vi "makeBlankPic.vi"(7 "File Path":path, 11 "previousImageData":T2) -> (1 "bottom":i16, 2 "right":i16, 3 "missingPicture":picture)   [LabVIEW 2022 SP3]
uses:
  <vilib>/picture/picture.llb/imagedata.ctl
  TOAPspecs.ctl
panel:
  in  "TOAPspecs":T1={"textOrigin"={"x"=0, "y"=0}, "textAlignment"={"horizontal"=enum."center", "vertical"=enum."center"}, "fontColour"={"text color"=16448250, "BG color"=1132933, "orientation "=enum."None"}, "fontChoice"=enum."User-specified Font", "userFont"={"Font Name:"="Courier New", "Size"=14, "Strikeout?"=FALSE, "Italic?"=FALSE, "Underline?"=FALSE, "Outline?"=FALSE, "Shadow?"=FALSE, "Bold?"=FALSE}}
  out "missingImageData":T2
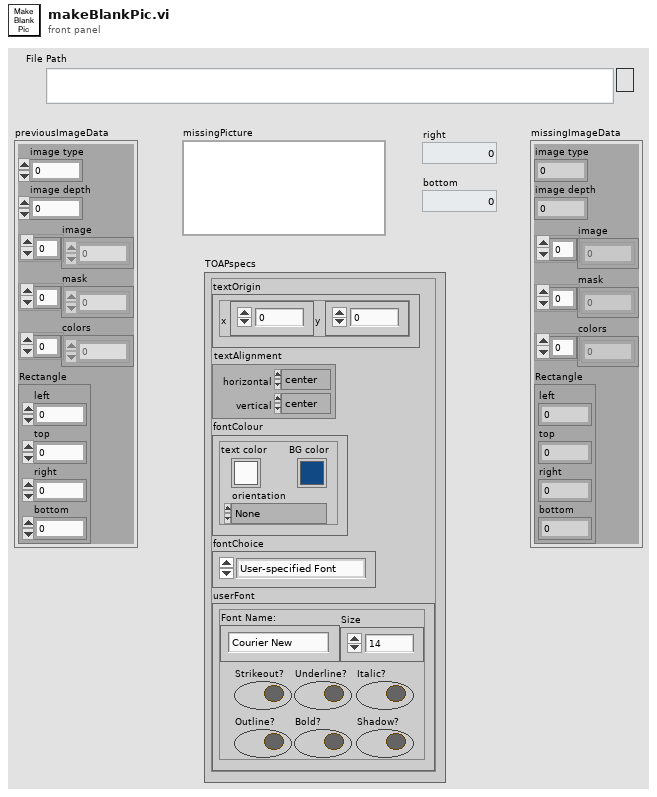
[diagram p1: front panel]
types:
  T1 = typedef "TOAPspecs.ctl" = cluster{"textOrigin":cluster{"x":i16, "y":i16}, "textAlignment":cluster{"horizontal":enum16{"left", "center", "right"}, "vertical":enum16{"top", "center", "bottom"}}, "fontColour":cluster{"text color":u32, "BG color":u32, "orientation ":enum16{"None", "Stacked", "Clockwise", "Counterclockwise"}}, "fontChoice":enum16{"User-specified Font", "Application Font", "System Font", "Dialog Font"}, "userFont":cluster{"Font Name:":string, "Size":i16, "Strikeout?":bool, "Italic?":bool, "Underline?":bool, "Outline?":bool, "Shadow?":bool, "Bold?":bool}}
  T2 = typedef "imagedata.ctl" = cluster{"image type":i32, "image depth":i32, "image":u8[], "mask":u8[], "colors":u32[], "Rectangle":cluster{"left":i16, "top":i16, "right":i16, "bottom":i16}}
  T3 = cluster{"Font Name:":string, "Size":i16, "Strikeout?":bool, "Italic?":bool, "Underline?":bool, "Outline?":bool, "Shadow?":bool, "Bold?":bool}
  T4 = enum16{"User-specified Font", "Application Font", "System Font", "Dialog Font"}
  T5 = cluster{"horizontal":enum16{"left", "center", "right"}, "vertical":enum16{"top", "center", "bottom"}}
  T6 = enum16{"None", "Stacked", "Clockwise", "Counterclockwise"}
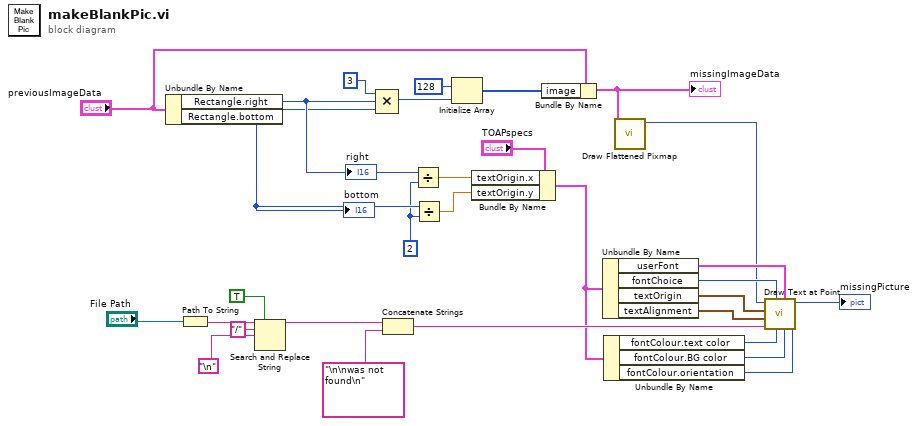
[diagram p0: block diagram]
diagram:
  w1 = i16 2 ("y")
  n1 = Unbundle By Name("previousImageData") -> ("Rectangle.right"=w4:i16, "Rectangle.bottom"=w3:i16)
  "bottom" <- w3
  "right" <- w4
  n2 = Path To String(path="File Path") -> (string=w10:string)
  n3 = Search and Replace String(replace all?=TRUE ("replace all? (F)"), input string=w10, search string="/", replace string="\n") -> (result string=w11:string)  [unwired: 4 in, 3 out]
  n4 = Compound Arithmetic op=MULTIPLY(3 ("value"), w4, w3) -> (w27:i32)
  n5 = Concatenate Strings(w11, "\n\nwas not found\n" ("string")) -> (w13:string)
  n6 = Divide(x=w4, y=w1) -> (x/y=w5:dbl)
  n7 = Divide(x=w3, y=w1) -> (x/y=w2:dbl)
  n8 = Initialize Array(u8 128 ("element"), w27) -> (w17:u8[])
  n9 = Bundle By Name(cluster="TOAPspecs", "textOrigin.x"=w5, "textOrigin.y"=w2) -> (w6:T1)
  n10 = Bundle By Name(cluster="previousImageData", "image"=w17) -> (w28:T2)
  "missingImageData" <- w28
  n11 = Unbundle By Name(w6) -> ("userFont"=w24:T3, "fontChoice"=w23:T4, "textOrigin"=w22:cluster{"x":i16, "y":i16}, "textAlignment"=w21:T5)
  n12 = Unbundle By Name(w6) -> ("fontColour.text color"=w20:u32, "fontColour.BG color"=w19:u32, "fontColour.orientation"=w18:T6)
  n13 = call <vilib>:"Draw Flattened Pixmap.vi"("image data"=w28) -> ("new picture"=w15:picture)  [unwired: 8 in]
  n14 = call <vilib>:"Draw Text at Point.vi"("text orientation"=w18, "BG color(transparent)"=w19, "[user-specified font]"=w24, "text color(black)"=w20, "desired font(Application)"=w23, "text"=w13, "alignment(left, top)"=w21, "origin"=w22, "picture"=w15) -> ("new picture"=→"missingPicture":picture)  [unwired: 1 in, 1 out]
